vi "Lab1_2.vi"() -> ()   [LabVIEW 2021]
panel:
  out "LED 3":bool
  out "LED 2":bool
  out "LED 1":bool
  in  "Sequence LED's":bool
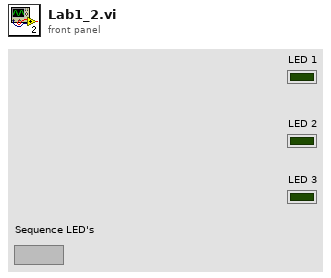
[diagram p1: front panel]
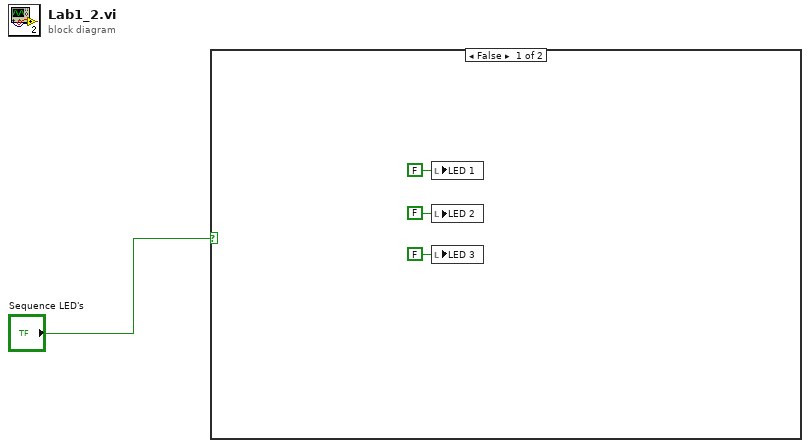
[diagram p0: block diagram]
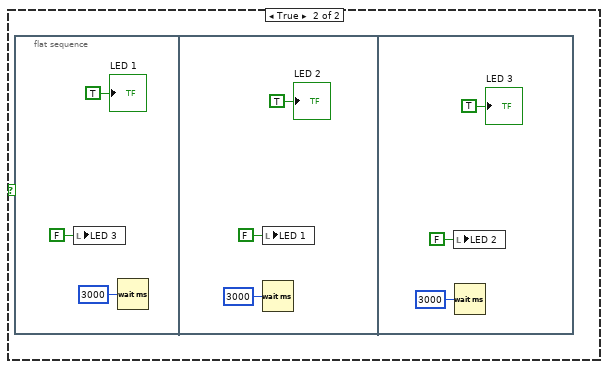
[diagram p2: hidden frame]
diagram:
  n1 = case shown="False" "Sequence LED's" {
    frame False {
      n2 = local write "LED 1"(FALSE ("LED 1")) -> ()
      n3 = local write "LED 2"(FALSE ("LED 2")) -> ()
      n4 = local write "LED 3"(FALSE ("LED 3")) -> ()
    }
    frame True {
      n5 = flat-sequence {
        frame #0 {
          n6 = local write "LED 3"(FALSE ("LED 3")) -> ()
          n7 = Wait (ms)(milliseconds to wait=u32 3000) -> ()  [unwired: 1 out]
          "LED 1" <- TRUE ("LED 1")
        }
        frame #1 {
          n8 = local write "LED 1"(FALSE ("LED 1")) -> ()
          n9 = Wait (ms)(milliseconds to wait=u32 3000) -> ()  [unwired: 1 out]
          "LED 2" <- TRUE ("LED 2")
        }
        frame #2 {
          n10 = local write "LED 2"(FALSE ("LED 2")) -> ()
          n11 = Wait (ms)(milliseconds to wait=u32 3000) -> ()  [unwired: 1 out]
          "LED 3" <- TRUE ("LED 3")
        }
      }
    }
  }
